vi "Stop Process.vi"(8 "error in (no error)":errorcluster, 11 "Main in":refnum<class "Main.lvclass">) -> (0 "error out":errorcluster, 3 "Main out":refnum<class "Main.lvclass">)   [LabVIEW 2019, in "Main.lvclass"]
doc: "Developed by Kevin Thompson\nkevin@thompsonengineering.net\n\nCopyright 2018\nThompson Engineering, LLC"
uses:
  Main.lvclass
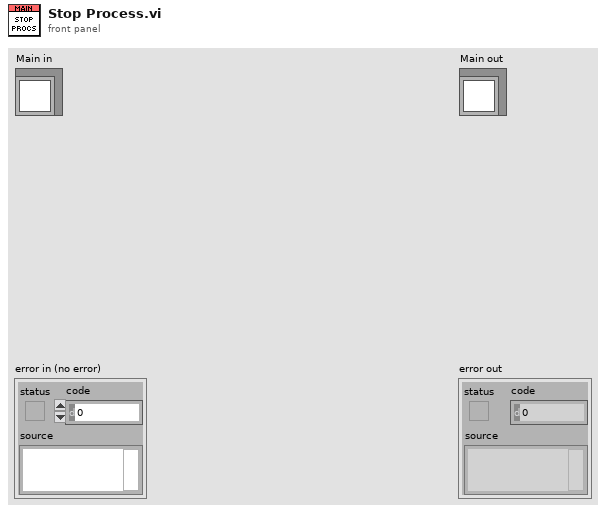
[diagram p1: front panel]
types:
  T1 = typedef "Main.lvclass/Public Events--cluster.ctl" = cluster{"Main.AsyncCmd Event":refnum<user-event>, "Main.AsyncMsg Event":refnum<user-event>, "stop process":refnum<user-event>, "UpdateControlValue Ev":refnum<user-event>, "ProcessingStateChg Ev":refnum<user-event>}
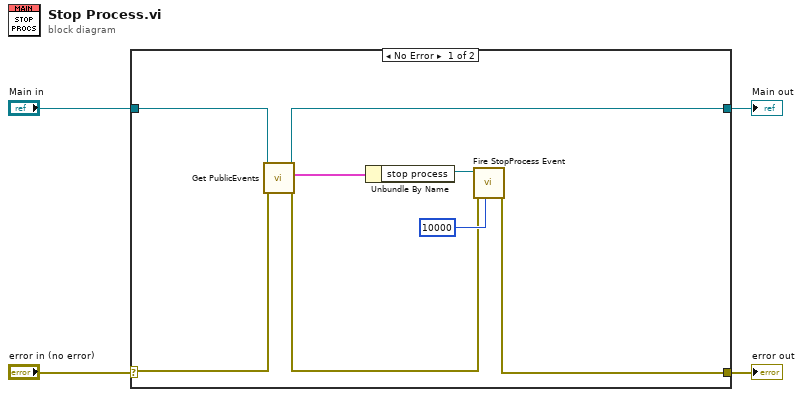
[diagram p0: block diagram]
diagram:
  n1 = case shown="No Error" "error in (no error)" {
    selector: "error in (no error)" -> [w6 w14]
    tunnel: [w12 w14] -> w3
    tunnel: [w8 w13] -> w1
    tunnel: "Main in" -> [w7 w13]
    frame No Error {
      n2 = call "Get PublicEvents.vi"("error in (no error)"=w6, "Main in"=w7) -> ("error out"=w5:errorcluster, "Public Events"=w9:T1, "Main out"=w8:refnum<class "Main.lvclass">)  [unwired: 7 in]
      n3 = Unbundle By Name(w9) -> ("stop process"=w11:refnum<user-event>)
      n4 = call "Fire StopProcess Event.vi"("timeout in ms (5000)"=10000, "error in (no error)"=w5, "Event in"=w11) -> ("error out"=w12:errorcluster)  [unwired: 5 in, 3 out]
    }
    frame Error {
    }
  }
  "error out" <- w3
  "Main out" <- w1
